vi "TH_Graphdata_To_Mean.vi"(6 "chart length (points)":i32, 7 "XY chart data":cluster{"x":dbl, "y":dbl}[](array[cluster]) {"y" format="%.2f"; "x" format="%.2f"}) -> (2 "ArraySize":i32, 3 "MeanValue":dbl format="%.1f")   [LabVIEW 2020]
uses:
  <vilib>/Analysis/baseanly.llb/Mean (DBL).vi
  <vilib>/Analysis/NI_AALBase.lvlib
panel:
  out "Y-Data":dbl[](array[numeric]) format="%.1f"
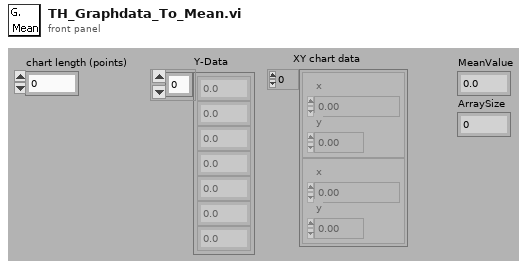
[diagram p1: front panel]
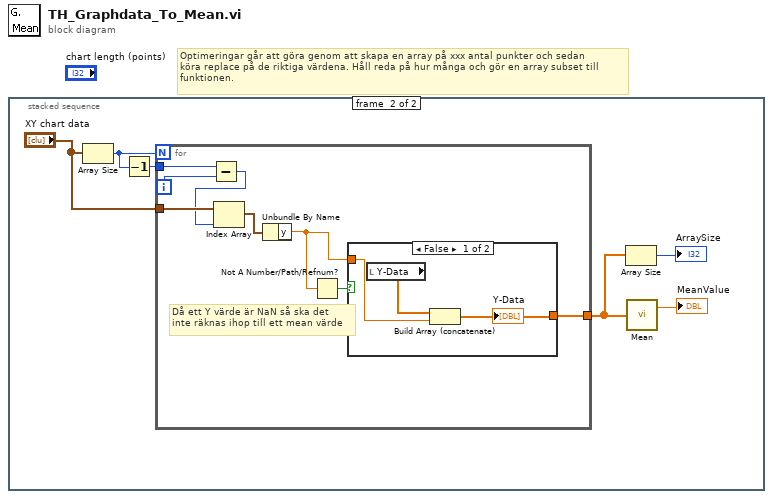
[diagram p0: block diagram]
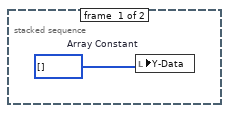
[diagram p2: hidden frame]
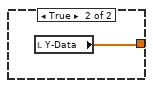
[diagram p3: hidden frame]
diagram:
  # "Optimeringar går att göra genom att skapa en array på xxx antal punkter och sedan\nköra replace på de riktiga värdena. Håll reda på hur många och gör en array subset till\nfunktionen."
  n1 = stacked-sequence {
    frame #0 {
      w1 = i32[] []  # Array Constant
      n2 = local write "Y-Data"(w1) -> ()
    }
    frame #1 {
      n3 = Array Size(array="XY chart data") -> (size(s)=w2:i32)
      n4 = Decrement(x=w2) -> (x-1=w3:i32)
      n5 = for {
        N: w2 -> [_]
        tunnel: "XY chart data" -> [w14]
        tunnel: [w15] -> w4
        tunnel: w3 -> [w10]
        i -> [w12]
        # "Då ett Y värde är NaN så ska det\ninte räknas ihop till ett mean värde"
        n6 = Subtract(x=w10, y=w12) -> (x-y=w11:i32)
        n7 = Index Array(array=w14, index=w11) -> (element=w13:cluster{"x":dbl, "y":dbl})
        n8 = Unbundle By Name(w13) -> ("y"=w9:dbl)
        n9 = Not A Number/Path/Refnum?(number/path/refnum=w9) -> (NaN/Path/Refnum?=w8:bool)
        n10 = case shown="False" w8 {
          tunnel: w9 -> [w16 _]
          tunnel: [w18 w19] -> w15
          frame False {
            n11 = local read "Y-Data"() -> (w17:dbl[])
            n12 = Build Array (concatenate)(w17, w16) -> (w18:dbl[])
            "Y-Data" <- w18
          }
          frame True {
            n13 = local read "Y-Data"() -> (w19:dbl[])
          }
        }
      }
      n14 = Array Size(array=w4) -> (size(s)=→"ArraySize":i32)
      n15 = call-poly <vilib>:"Mean.vi"("X"=w4) -> ("mean"=→"MeanValue":dbl)  [unwired: 1 out]
    }
  }
